vi "MultiAxisDemo.vi"() -> ()   [LabVIEW 2010]
doc: "Demo application used for the PUMA 560. Control and read out for all six axes. Ability to read in target positions in encoder counts, joint angle in degrees, and joint angle in radians from a tab delimited text file, and save them back to a file. Ability to specify trajectory acceleration and velocity in encoder counts, radians, and degrees.\n\nDependencies:\n\nSubVIs:\n\nCheck for Kill.vi\nCheck Start Move.vi\nCheck Find Home.vi\nLoad Joint Angle.vi\nLoad Joint Velocity.vi\nLoad Joint Acceleration.vi\nRead Pot.vi\nRead Joint Angle.vi\nRead Joint Velocity.vi\nRead Joint Config.vi\nsingleAxisMultiMove.vi\nfindHome_Puma560.vi\n\nTypedefs:\n\nPosition Mode.ctl\nTrajectory Parameters.ctl\nControls.ctl"
uses:
  Shared/typedefs/Trajectory Parameters.ctl
  Typedefs/Units_Enum.ctl
  Typedefs/AxisSpaceControls_ClusterofAxisControls.ctl
  Typedefs/AxisControls_cluster.ctl
  <vilib>/Motion/FlexMotion/CustomControls/CustomControls.llb/Axis To Control.flx
  Typedefs/AxisSpaceIndicator_ArrayofAxisIndicator.ctl
  Typedefs/AxisIndicator_cluster.ctl
  <vilib>/Utility/file.llb/Write To Spreadsheet File (I64).vi
  <vilib>/Utility/file.llb/Read From Spreadsheet File (I64).vi
panel:
  in  "Axis Cfg":bool
  out "Indicators":T1=[{"Pot Value"=2.6260421911955447, "Joint Angle"=0.0, "Software Limit"=FALSE, "Following Error Limit"=FALSE, "Move Complete"=TRUE, "Motor Killed"=FALSE, "Joint Velocity"=0.0, "Following Error"=0}, {"Pot Value"=2.3157499809262228, "Joint Angle"=0.0, "Software Limit"=FALSE, "Following Error Limit"=FALSE, "Move Complete"=TRUE, "Motor Killed"=FALSE, "Joint Velocity"=0.0, "Following Error"=0}, {"Pot Value"=1.879189364461738, "Joint Angle"=0.0, "Software Limit"=FALSE, "Following Error Limit"=FALSE, "Move Complete"=TRUE, "Motor Killed"=FALSE, "Joint Velocity"=0.0, "Following Error"=0}, {"Pot Value"=2.2236617837796597, "Joint Angle"=0.0, "Software Limit"=FALSE, "Following Error Limit"=FALSE, "Move Complete"=TRUE, "Motor Killed"=FALSE, "Joint Velocity"=0.0, "Following Error"=0}, {"Pot Value"=3.769476997024491, "Joint Angle"=0.015016058840704642, "Software Limit"=FALSE, "Following Error Limit"=FALSE, "Move Complete"=TRUE, "Motor Killed"=FALSE, "Joint Velocity"=0.0, "Following Error"=0}, {"Pot Value"=2.4994686045624475, "Joint Angle"=-0.004694468351459197, "Software Limit"=FALSE, "Following Error Limit"=FALSE, "Move Complete"=TRUE, "Motor Killed"=FALSE, "Joint Velocity"=0.0, "Following Error"=0}] {"Joint Velocity" format="%#_4g"; "Joint Angle" format="%#_4g"; "Pot Value" format="%#_4g"}
  in  "Controls":T3={"Axis 1"={"Axis"=1, "Enable"=TRUE, "Start"=FALSE, "Home"=FALSE, "Stop Type"=0, "Kill"=FALSE}, "Axis 2"={"Axis"=2, "Enable"=TRUE, "Start"=FALSE, "Home"=FALSE, "Stop Type"=0, "Kill"=FALSE}, "Axis 3"={"Axis"=3, "Enable"=TRUE, "Start"=FALSE, "Home"=FALSE, "Stop Type"=0, "Kill"=FALSE}, "Axis 4"={"Axis"=4, "Enable"=TRUE, "Start"=FALSE, "Home"=FALSE, "Stop Type"=0, "Kill"=FALSE}, "Axis 5"={"Axis"=5, "Enable"=FALSE, "Start"=FALSE, "Home"=FALSE, "Stop Type"=0, "Kill"=FALSE}, "Axis 6"={"Axis"=6, "Enable"=FALSE, "Start"=FALSE, "Home"=FALSE, "Stop Type"=0, "Kill"=FALSE}} {"Axis 6"."Stop Type" items=["Decelerate", "Halt", "Kill"]; "Axis 6"."Axis" items=["Axis 1"=1, "Axis 2"=2, "Axis 3"=3, "Axis 4"=4, "Axis 5"=5, "Axis 6"=6, "Axis 7"=7, "Axis 8"=8]; "Axis 5"."Stop Type" items=["Decelerate", "Halt", "Kill"]; "Axis 5"."Axis" items=["Axis 1"=1, "Axis 2"=2, "Axis 3"=3, "Axis 4"=4, "Axis 5"=5, "Axis 6"=6, "Axis 7"=7, "Axis 8"=8]; "Axis 4"."Stop Type" items=["Decelerate", "Halt", "Kill"]; "Axis 4"."Axis" items=["Axis 1"=1, "Axis 2"=2, "Axis 3"=3, "Axis 4"=4, "Axis 5"=5, "Axis 6"=6, "Axis 7"=7, "Axis 8"=8]; "Axis 3"."Stop Type" items=["Decelerate", "Halt", "Kill"]; "Axis 3"."Axis" items=["Axis 1"=1, "Axis 2"=2, "Axis 3"=3, "Axis 4"=4, "Axis 5"=5, "Axis 6"=6, "Axis 7"=7, "Axis 8"=8]; "Axis 2"."Stop Type" items=["Decelerate", "Halt", "Kill"]; "Axis 2"."Axis" items=["Axis 1"=1, "Axis 2"=2, "Axis 3"=3, "Axis 4"=4, "Axis 5"=5, "Axis 6"=6, "Axis 7"=7, "Axis 8"=8]; "Axis 1"."Stop Type" items=["Decelerate", "Halt", "Kill"]; "Axis 1"."Axis" items=["Axis 1"=1, "Axis 2"=2, "Axis 3"=3, "Axis 4"=4, "Axis 5"=5, "Axis 6"=6, "Axis 7"=7, "Axis 8"=8]}
  in  "Target Positions":i32[][](array[numeric])=[[45, 45, 45, 45, 0, 0]]
  in  "Unit Mode":T6=enum."Degrees"
  in  "Target Position File Path":path
  in  "Save":bool
  in  "Load":bool
  in  "Stop Type":u16(ring) items=["Decelerate", "Halt", "Kill"]
  in  "Board ID":T7=1 min=1 max=32 step=1
  in  "Trajectory Parameters":T8={"Operation Mode (Absolute)"=0, "Blend"=FALSE, "Velocity"=6.0, "Acceleration"=4.0, "Deceleration"=4.0, "Blend Factor"=0, "Permitted Following Error"=1000.0, "S Curve Time"=0} {"Operation Mode (Absolute)" items=["Absolute Position", "Relative Position"]; "Velocity" min=0.0 max=500.0 step=1.0}
  in  "Run Mode":enum32{"Sequential", "Parallel"}(radio)=enum."Parallel"
  in  "Home All":bool
  in  "Kill All":bool
  in  "End Program":bool
  in  "Start All":bool
  # "NOTE : Please set Board ID before executing program"
  # "Change gear ratios, counts/revolution, etc."
  # "Axis 1"
  # "Axis 2"
  # "Axis 3"
  # "Axis 4"
  # "Axis 5"
  # "Axis 6"
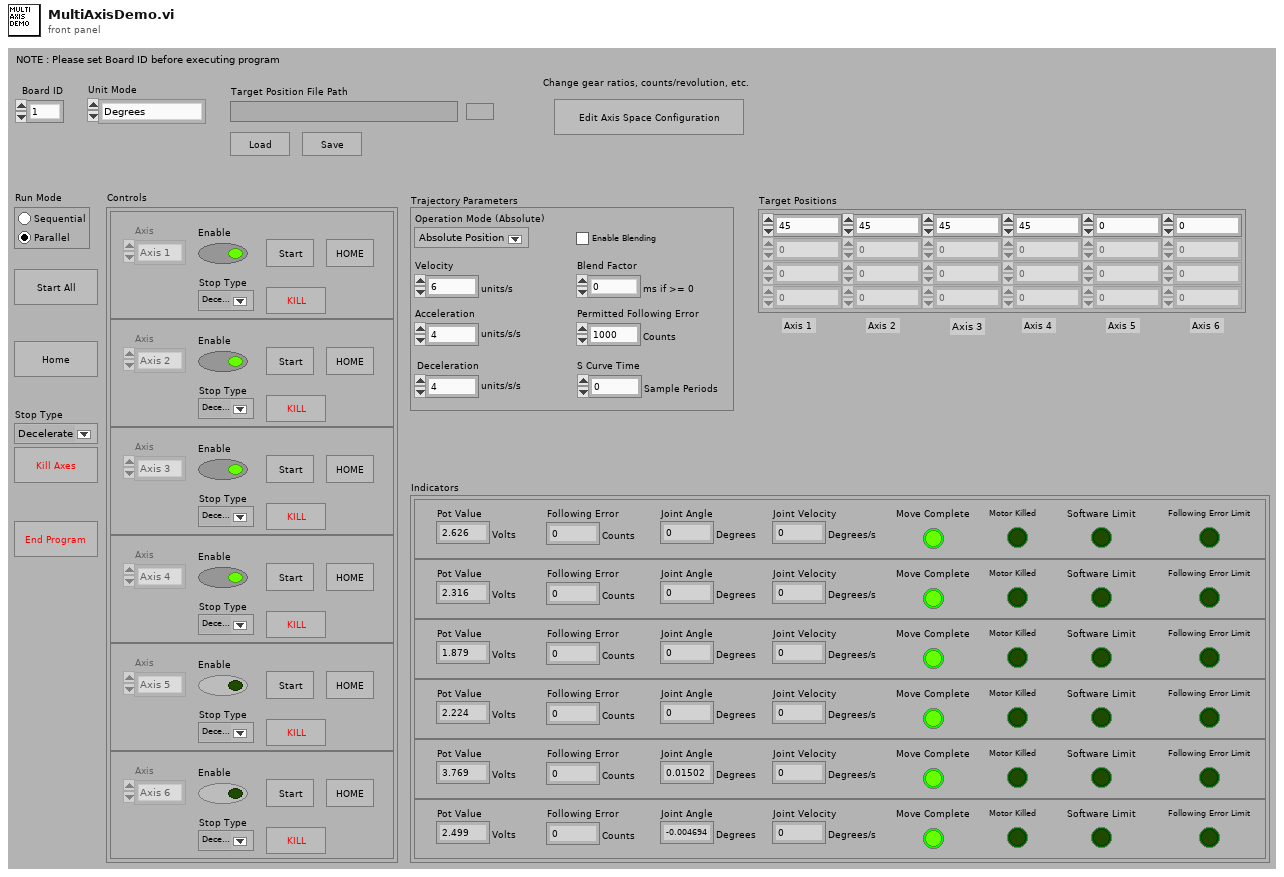
[diagram p1: front panel]
types:
  T1 = typedef "AxisSpaceIndicator_ArrayofAxisIndicator.ctl" = T2[]
  T2 = typedef "AxisIndicator_cluster.ctl" = cluster{"Pot Value":dbl, "Joint Angle":dbl, "Software Limit":bool, "Following Error Limit":bool, "Move Complete":bool, "Motor Killed":bool, "Joint Velocity":dbl, "Following Error":i16}
  T3 = typedef "AxisSpaceControls_ClusterofAxisControls.ctl" = cluster{"Axis 1":T4, "Axis 2":T4, "Axis 3":T4, "Axis 4":T4, "Axis 5":T4, "Axis 6":T4}
  T4 = typedef "AxisControls_cluster.ctl" = cluster{"Axis":T5, "Enable":bool, "Start":bool, "Home":bool, "Stop Type":u16, "Kill":bool}
  T5 = typedef "Axis To Control.flx" = u16
  T6 = typedef "Units_Enum.ctl" = enum16{"Radians", "Encoder Counts", "Revolutions", "Degrees"}
  T7 = typedef "Board Id" = u8
  T8 = typedef "Trajectory Parameters.ctl" = cluster{"Operation Mode (Absolute)":u16, "Blend":bool, "Velocity":dbl, "Acceleration":dbl, "Deceleration":dbl, "Blend Factor":i16, "Permitted Following Error":dbl, "S Curve Time":u16}
  T9 = typedef "Bd Id Out" = u8
  T10 = cluster{"Ready to Receive":bool, "Return Data Pending":bool, "Reserved":bool, "CIP":bool, "Packet Error":bool, "Power Up Reset":bool, "Error Message":bool, "Hardware Fail":bool}
  T11 = typedef "Resource Out (Enum).flx" = u16
  T12 = cluster{"Run/Stop":bool, "Profile Complete":bool, "Motor Off ":bool, "Following Error":bool, "Limit Switch":bool, "Home Switch":bool, "SW Limit Switch":bool, "Watchdog":bool, "Velocity Threshold":bool, "Position Brkpt":bool, "Home Found":bool, "Index Found":bool, "High Speed Capture":bool, "Reverse Direction":bool, "Blend Complete":bool, "Move Complete":bool}
  T13 = cluster{"Axis 1":T4, "Axis 2":T4, "Axis 3":T4, "Axis 4":T4, "Axis 5":T4, "Axis 6":T4}
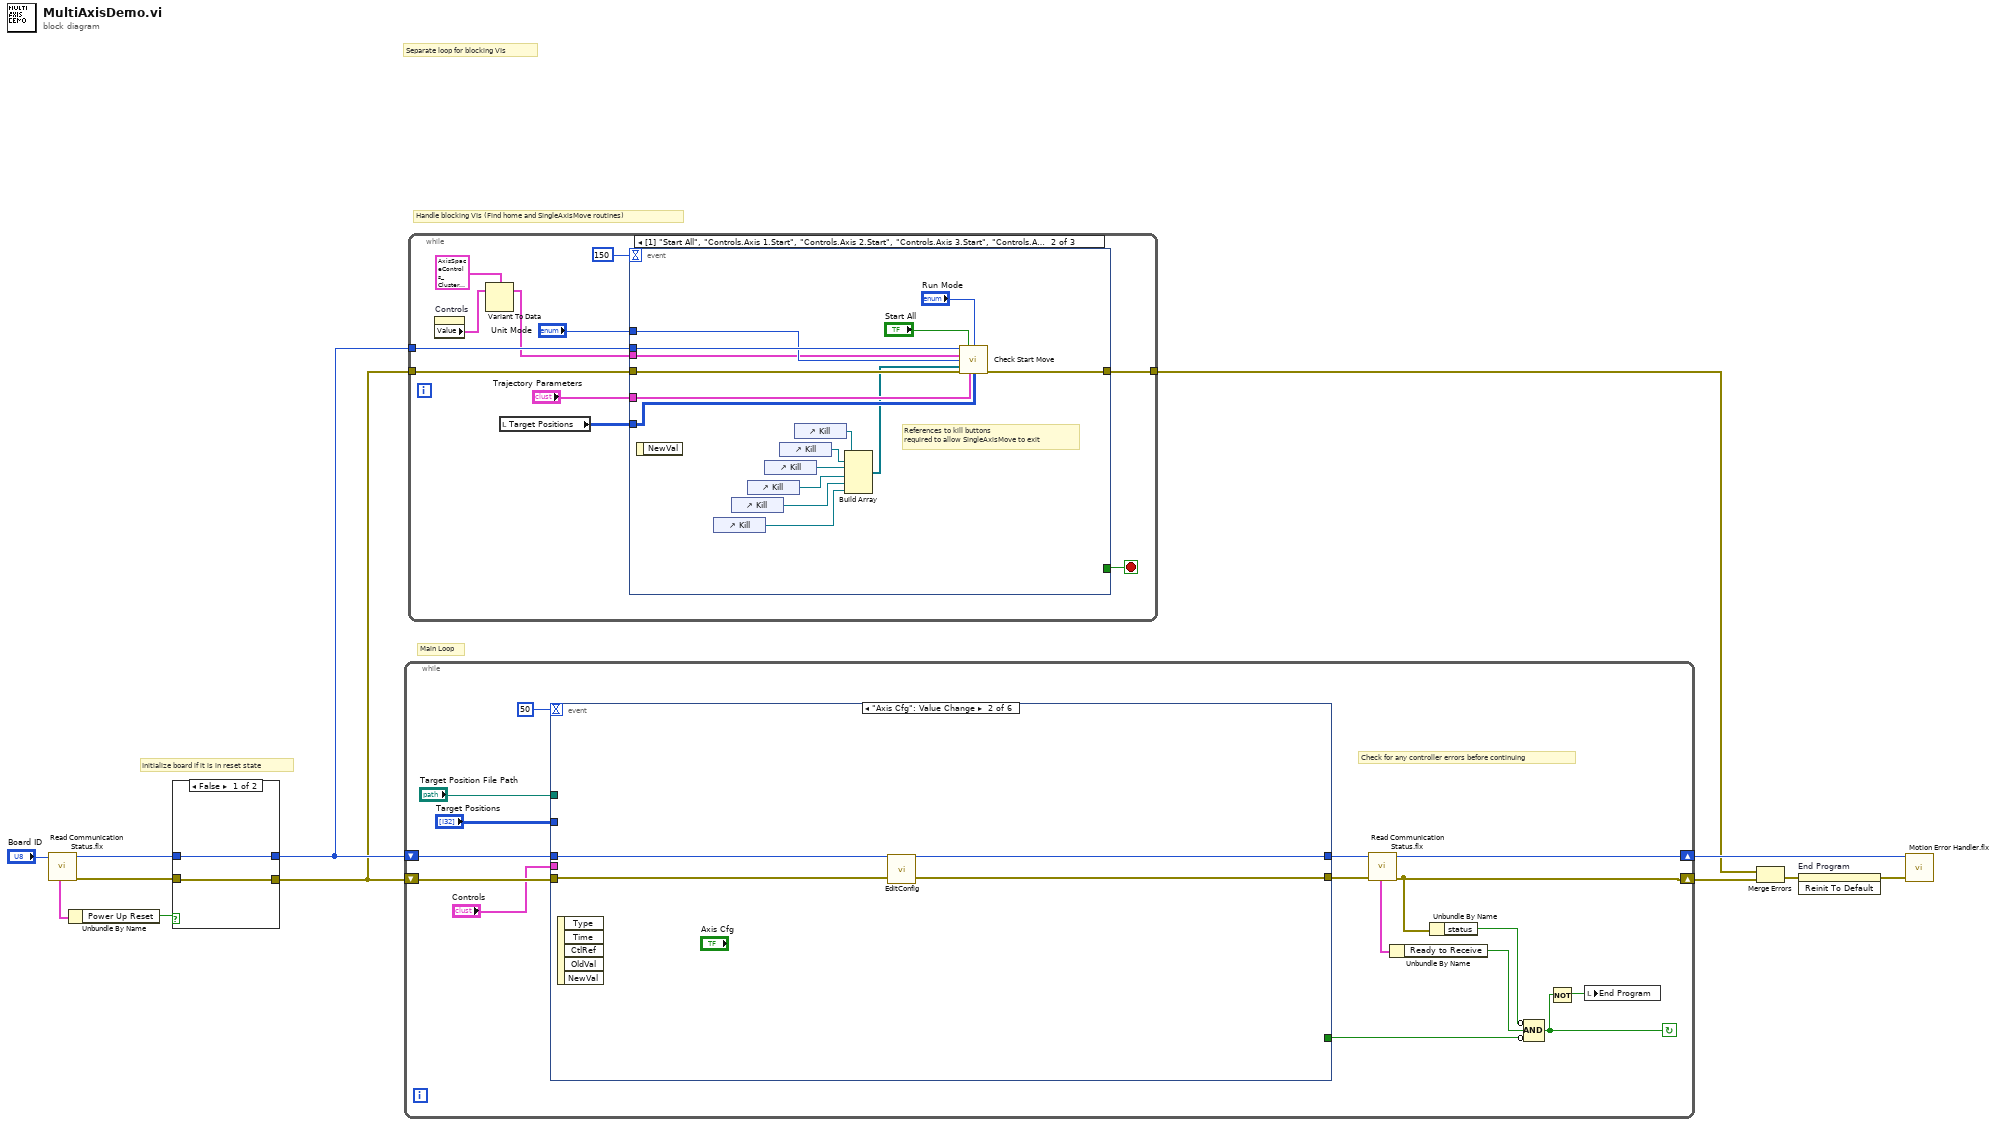
[diagram p0: block diagram]
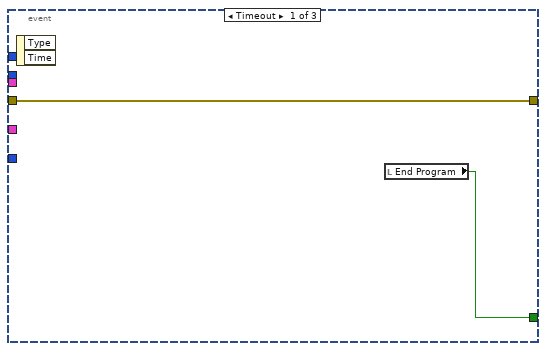
[diagram p2: hidden frame]
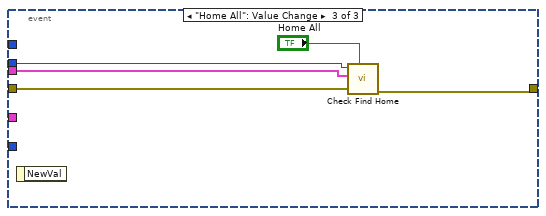
[diagram p3: hidden frame]
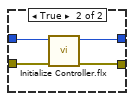
[diagram p4: hidden frame]
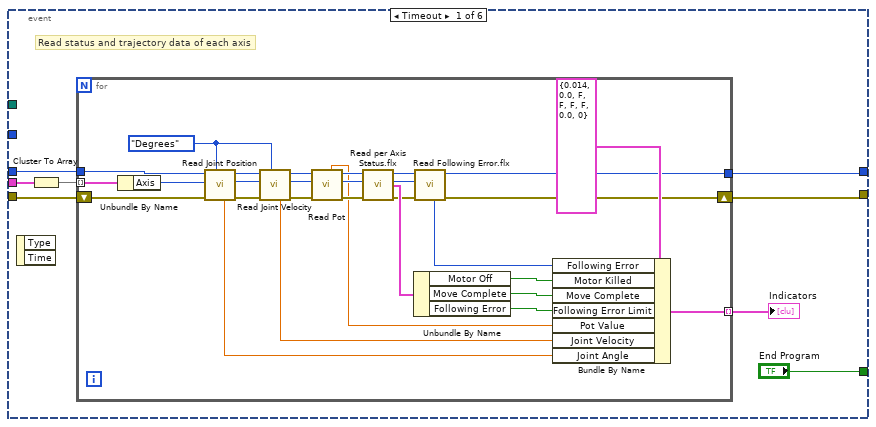
[diagram p5: hidden frame]
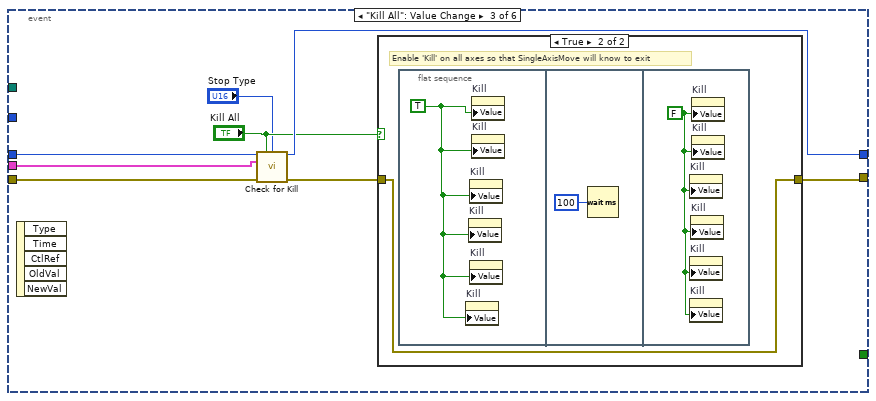
[diagram p6: hidden frame]
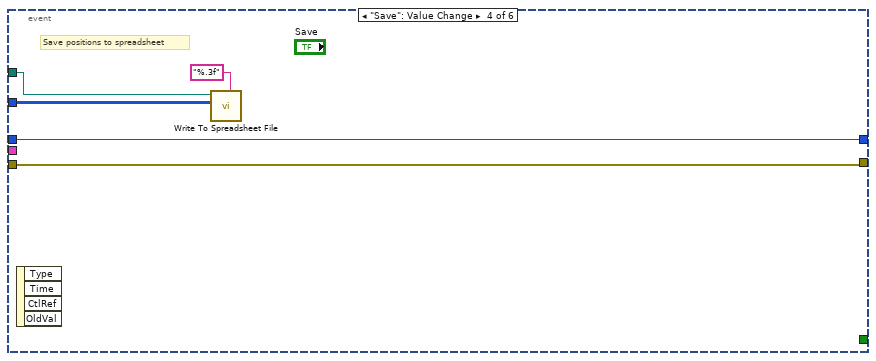
[diagram p8: hidden frame]
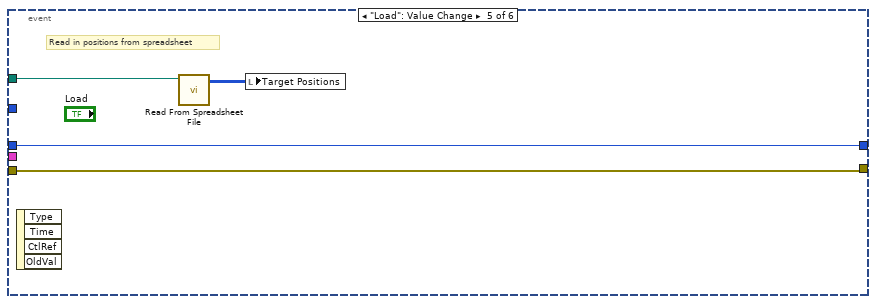
[diagram p9: hidden frame]
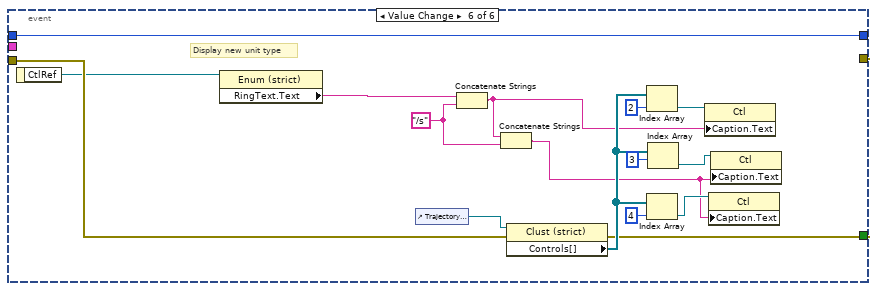
[diagram p10: hidden frame]
diagram:
  # "Handle blocking VIs (Find home and SingleAxisMove routines)"
  # "Separate loop for blocking VIs"
  # "Main Loop"
  # "Initialize board if it is in reset state"
  n1 = call <vilib>:"Read Communication Status.flx"("Board ID"="Board ID") -> ("error out"=w8:errorcluster, "Bd ID Out"=w11:T9, "Communication Status Register"=w10:T10)  [unwired: 5 in]
  n2 = Unbundle By Name(w10) -> ("Power Up Reset"=w9:bool)
  n3 = case shown="False" w9 {
    tunnel: [w14 w16] -> w5
    tunnel: w11 -> [w14 w17]
    tunnel: w8 -> [w13 w18]
    tunnel: [w13 w15] -> w4
    frame False {
    }
    frame True {
      n4 = call <vilib>:"Initialize Controller.flx"("error in (no error)"=w18, "Board ID"=w17) -> ("error out"=w15:errorcluster, "Bd ID Out"=w16:T9)  [unwired: 6 in]
    }
  }
  n5 = while {
    shift-right: [w31] -> w12
    shift-left: w4 -> [w33]
    shift-right: [w28] -> w6
    shift-left: w5 -> [w34]
    stop <- w32 continue-if-true
    # "Check for any controller errors before continuing"
    n6 = event shown="[1] \"Axis Cfg\": Value Change" {
      selector: _ -> [_ _ _ _ _ _]
      dyn-events: _ -> [_ _ _ _ _ _]
      timeout: 50 -> [_ _ _ _ _ _]
      tunnel: "Target Position File Path" -> [_ _ _ w92 w96 _]
      tunnel: w34 -> [w42 w73 w81 w91 w94 w112]
      tunnel: w33 -> [w41 w72 w82 w90 w95 w103]
      tunnel: [w40 w74 w75 w90 w95 w102] -> w29
      tunnel: [w39 w73 w79 w91 w94 w112] -> w30
      tunnel: "Target Positions" -> [_ _ _ w89 _ _]
      tunnel: "Controls" -> [w36 _ w80 _ _ _]
      tunnel: ["End Program" _ _ _ _ _] -> w27
      event Timeout {
        # "Read status and trajectory data of each axis"
        n7 = event-data() -> ()  [unwired: 1 in, 2 out]
        n8 = Cluster To Array(cluster=w36) -> (array=w37:T4[])
        n9 = for {
          tunnel: w42 -> [w67]
          tunnel: [w61] -> w38 mode=indexing
          shift-right: [w53] -> w40
          shift-left: w41 -> [w66]
          tunnel: w37 -> [w51] mode=indexing
          tunnel: [w50] -> w39
          w54 = Units_Enum."Degrees" ("Units (Encoder Counts)")
          n10 = Unbundle By Name(w51) -> ("Axis"=w52:T5)
          n11 = call "Read Joint Position.vi"("Units (Encoder Counts)"=w54, "error in (no error)"=w66, "Axis"=w52, "Board ID"=w67) -> ("error out"=w58:errorcluster, "Resource Output"=w59:T11, "Bd ID Out"=w60:T9, "Joint Position"=w43:dbl)  [unwired: 4 in]
          n12 = call "Read Joint Velocity.vi"("Units (Degrees)"=w54, "error in (no error)"=w58, "Axis"=w59, "Board ID"=w60) -> ("error out"=w57:errorcluster, "Resource Output"=w56:T11, "Bd ID Out"=w55:T9, "Joint Velocity"=w44:dbl)  [unwired: 4 in]
          n13 = call "Read Pot.vi"("error in (no error)"=w57, "Axis In"=w56, "Board ID"=w55) -> ("error out"=w71:errorcluster, "Axis Out"=w68:T5, "Bd ID Out"=w69:T9, "Pot Voltage"=w45:dbl)  [unwired: 5 in]
          n14 = call <vilib>:"Read per Axis Status.flx"("error in (no error)"=w71, "Axis"=w68, "Board ID"=w69) -> ("error out"=w65:errorcluster, "Resource Output"=w63:T11, "Bd ID Out"=w64:T9, "Per Axis H/W Status"=w70:T12)  [unwired: 3 in]
          n15 = Unbundle By Name(w70) -> ("Motor Off"=w49:bool, "Move Complete"=w48:bool, "Following Error"=w47:bool)
          n16 = call <vilib>:"Read Following Error.flx"("error in (no error)"=w65, "Axis or Vector Space"=w63, "Board Id"=w64) -> ("error out"=w53:errorcluster, "Bd Id Out"=w50:T9, "Following Error"=w46:i16)  [unwired: 3 in, 1 out]
          n17 = Bundle By Name(cluster=T2 {"Pot Value"=0.014, "Joint Angle"=0.0, "Software Limit"=FALSE, "Following Error Limit"=FALSE, "Move Complete"=FALSE, "Motor Killed"=FALSE, "Joint Velocity"=0.0, "Following Error"=0} ("Axis 1"), "Following Error"=w46, "Motor Killed"=w49, "Move Complete"=w48, "Following Error Limit"=w47, "Pot Value"=w45, "Joint Velocity"=w44, "Joint Angle"=w43) -> (w61:T2)
        }
        "Indicators" <- w38
      }
      event "Axis Cfg": Value Change {
        n18 = event-data() -> ()  [unwired: 1 in, 5 out]
        n19 = call "EditConfig.vi"("error in"=w72) -> ("error out"=w74:errorcluster)  [unwired: 1 in, 1 out]
      }
      event "Kill All": Value Change {
        n20 = event-data() -> ()  [unwired: 1 in, 5 out]
        n21 = call "Check for Kill.vi"("Bd ID In"=w81, "Kill All"="Kill All", "Stop Type"="Stop Type", "Controls"=w80, "error in"=w82) -> ("Bd ID Out"=w79:T9, "error out"=w76:errorcluster)  [unwired: 9 in]
        n22 = case shown="True" "Kill All" {
          tunnel: w76 -> [w83 w84]
          tunnel: [w83 w84] -> w75
          frame False {
          }
          frame True {
            # "Enable 'Kill' on all axes so that SingleAxisMove will know to exit"
            n23 = flat-sequence {
              frame #0 {
                w85 = TRUE ("Value")
                n24 = property on="Kill" class="Bool (strict)"("Value"=w85) -> ()  [unwired: 2 in, 2 out]
                n25 = property on="Kill" class="Bool (strict)"("Value"=w85) -> ()  [unwired: 2 in, 2 out]
                n26 = property on="Kill" class="Bool (strict)"("Value"=w85) -> ()  [unwired: 2 in, 2 out]
                n27 = property on="Kill" class="Bool (strict)"("Value"=w85) -> ()  [unwired: 2 in, 2 out]
                n28 = property on="Kill" class="Bool (strict)"("Value"=w85) -> ()  [unwired: 2 in, 2 out]
                n29 = property on="Kill" class="Bool (strict)"("Value"=w85) -> ()  [unwired: 2 in, 2 out]
              }
              frame #1 {
                n30 = Wait (ms)(milliseconds to wait=u32 100) -> ()  [unwired: 1 out]
              }
              frame #2 {
                w87 = FALSE ("Value")
                n31 = property on="Kill" class="Bool (strict)"("Value"=w87) -> ()  [unwired: 2 in, 2 out]
                n32 = property on="Kill" class="Bool (strict)"("Value"=w87) -> ()  [unwired: 2 in, 2 out]
                n33 = property on="Kill" class="Bool (strict)"("Value"=w87) -> ()  [unwired: 2 in, 2 out]
                n34 = property on="Kill" class="Bool (strict)"("Value"=w87) -> ()  [unwired: 2 in, 2 out]
                n35 = property on="Kill" class="Bool (strict)"("Value"=w87) -> ()  [unwired: 2 in, 2 out]
                n36 = property on="Kill" class="Bool (strict)"("Value"=w87) -> ()  [unwired: 2 in, 2 out]
              }
            }
          }
        }
      }
      event "Save": Value Change {
        # "Save positions to spreadsheet"
        n37 = event-data() -> ()  [unwired: 1 in, 4 out]
        n38 = call-poly <vilib>:"Write To Spreadsheet File.vi"("format (%d)"="%.3f" ("format (%.3f)"), "2D data"=w89, "file path (dialog if empty)"=w92) -> ()  [unwired: 5 in, 1 out]
      }
      event "Load": Value Change {
        # "Read in positions from spreadsheet"
        n39 = event-data() -> ()  [unwired: 1 in, 4 out]
        n40 = call-poly <vilib>:"Read From Spreadsheet File.vi"("file path (dialog if empty)"=w96) -> ("all rows"=w93:i64[][])  [unwired: 6 in, 4 out]
        n41 = local write "Target Positions"(w93) -> ()
      }
      event Value Change {
        w99 = "/s" ("string")
        # "Display new unit type"
        n42 = event-data() -> ("CtlRef"=w98:refnum<vi>)  [unwired: 1 in]
        n43 = property class="Enum (strict)"(reference=w98) -> ("RingText.Text"=w97:string)  [unwired: 1 in, 2 out]
        n44 = control-ref of="Trajectory Parameters"() -> (w104:refnum<vi>)
        n45 = Concatenate Strings(w97, w99) -> (w100:string)
        n46 = Concatenate Strings(w100, w99) -> (w101:string)
        n47 = property class="Clust (strict)"(reference=w104, error in=w103) -> (error out=w102:errorcluster, "Controls[]"=w109:refnum<vi>[])  [unwired: 1 out]
        n48 = Index Array(array=w109, index=2) -> (element=w107:refnum<vi>)
        n49 = Index Array(array=w109, index=4) -> (element=w111:refnum<vi>)
        n50 = Index Array(array=w109, index=3) -> (element=w108:refnum<vi>)
        n51 = property class="Ctl"(reference=w107, "Caption.Text"=w100) -> ()  [unwired: 1 in, 2 out]
        n52 = property class="Ctl"(reference=w111, "Caption.Text"=w101) -> ()  [unwired: 1 in, 2 out]
        n53 = property class="Ctl"(reference=w108, "Caption.Text"=w101) -> ()  [unwired: 1 in, 2 out]
      }
    }
    n54 = call <vilib>:"Read Communication Status.flx"("error in (no error)"=w29, "Board ID"=w30) -> ("error out"=w31:errorcluster, "Bd ID Out"=w28:T9, "Communication Status Register"=w19:T10)  [unwired: 4 in]
    n55 = Unbundle By Name(w19) -> ("Ready to Receive"=w21:bool)
    n56 = Unbundle By Name(w31) -> ("status"=w20:bool)
    n57 = Compound Arithmetic op=AND(invert w20, w21, invert w27) -> (w32:bool)
    n58 = Not(x=w32) -> (.not. x?=w22:bool)
    n59 = local write "End Program"(w22) -> ()
  }
  n60 = while {
    tunnel: w5 -> [w123]
    tunnel: w4 -> [w122]
    tunnel: [w117] -> w3
    stop <- w116 stop-if-true
    n61 = property on="Controls" class="Clust (strict)"() -> ("Value"=w114:T13)  [unwired: 2 in, 2 out]
    n62 = Variant To Data(Variant=w114, type=T3 {"Axis 1"={"Axis"=1, "Enable"=FALSE, "Start"=FALSE, "Home"=FALSE, "Stop Type"=0, "Kill"=FALSE}, "Axis 2"={"Axis"=1, "Enable"=FALSE, "Start"=FALSE, "Home"=FALSE, "Stop Type"=0, "Kill"=FALSE}, "Axis 3"={"Axis"=1, "Enable"=FALSE, "Start"=FALSE, "Home"=FALSE, "Stop Type"=0, "Kill"=FALSE}, "Axis 4"={"Axis"=1, "Enable"=FALSE, "Start"=FALSE, "Home"=FALSE, "Stop Type"=0, "Kill"=FALSE}, "Axis 5"={"Axis"=1, "Enable"=FALSE, "Start"=FALSE, "Home"=FALSE, "Stop Type"=0, "Kill"=FALSE}, "Axis 6"={"Axis"=1, "Enable"=FALSE, "Start"=FALSE, "Home"=FALSE, "Stop Type"=0, "Kill"=FALSE}} ("Axis Controls")) -> (data=w113:T3)  [unwired: 1 in, 1 out]
    n63 = local read "Target Positions"() -> (w121:i32[][])
    n64 = event shown="[1] \"Start All\", \"Controls.Axis 1.Start\", \"Controls.Axis 2.Start\", \"Controls.Axis 3.Start\", \"Controls.Axis 4.Start\", \"Controls.Axis 5.Start\", \"Controls.Axis 6.Start\": Value Change" {
      selector: _ -> [_ _ _]
      dyn-events: _ -> [_ _ _]
      timeout: 150 -> [_ _ _]
      tunnel: w123 -> [_ w141 w146]
      tunnel: w122 -> [w125 w140 w144]
      tunnel: [w125 w139 w143] -> w117
      tunnel: w121 -> [_ w138 _]
      tunnel: "Unit Mode" -> [_ w137 _]
      tunnel: "Trajectory Parameters" -> [_ w136 _]
      tunnel: w113 -> [_ w128 w142]
      tunnel: [w124 _ _] -> w116
      event Timeout {
        n65 = event-data() -> ()  [unwired: 1 in, 2 out]
        n66 = local read "End Program"() -> (w124:bool)
      }
      event "Start All": Value Change {
        # "References to kill buttons\nrequired to allow SingleAxisMove to exit"
        n67 = event-data() -> ()  [unwired: 1 in, 1 out]
        n68 = control-ref of="Kill"() -> (w133:refnum<vi>)
        n69 = control-ref of="Kill"() -> (w132:refnum<vi>)
        n70 = control-ref of="Kill"() -> (w131:refnum<vi>)
        n71 = control-ref of="Kill"() -> (w130:refnum<vi>)
        n72 = control-ref of="Kill"() -> (w129:refnum<vi>)
        n73 = control-ref of="Kill"() -> (w126:refnum<vi>)
        n74 = Build Array(w126, w129, w130, w131, w132, w133) -> (w127:refnum<vi>[])
        n75 = call "Check Start Move.vi"("Bd ID In"=w141, "Start All (False)"="Start All", "Run Mode"="Run Mode", "Axis Controls"=w128, "Units (Encoder Counts)"=w137, "Stop refnum array"=w127, "error in"=w140, "Trajectory Parameters"=w136, "Target Positions"=w138) -> ("error out"=w139:errorcluster)  [unwired: 5 in, 1 out]
      }
      event "Home All": Value Change {
        n76 = event-data() -> ()  [unwired: 1 in, 1 out]
        n77 = call "Check Find Home.vi"("Home All"="Home All", "error in"=w144, "Controls"=w142, "Bd ID In"=w146) -> ("error out"=w143:errorcluster)  [unwired: 6 in, 1 out]
      }
    }
  }
  n78 = Merge Errors(w3, w12) -> (w2:errorcluster)
  n79 = invoke on="End Program" class="Bool (strict)" method="Reinit To Default"(error in=w2) -> (error out=w1:errorcluster)  [unwired: 2 in, 2 out]
  n80 = call <vilib>:"Motion Error Handler.flx"("Board ID"=w6, "error in (no error)"=w1) -> ()  [unwired: 9 in, 5 out]
